vi "GeoData.vi"() -> ()   [LabVIEW 2017] (continued)
County\tH1\n52577\t19123\tOskaloosa\tIA\tMahaska County\tH1\n50256\t19123\tTracy\tIA\tMahaska County\tH1\n52595\t19123\tUniversity park\tIA\tMahaska County\tH1\n50207\t19123\tNew sharon\tIA\tMahaska County\tH1\n50027\t19123\tBarnes city\tIA\tMahaska County\tH1\n50170\t19125\tMonroe\tIA\tMarion County\tH1\n50163\t19125\tMelcher dallas\tIA\tMarion County\tH1\n50049\t19125\tChariton\tIA\tMarion County\tH1\n50138\t19125\tKnoxville\tIA\tMarion County\tH1\n50219\t19125\tPella\tIA\tMarion County\tH1\n50214\t19125\tOtley\tIA\tMarion County\tH1\n50143\t19125\tLeighton\tIA\tMarion County\tH1\n50237\t19125\tRunnells\tIA\tMarion County\tH1\n50252\t19125\tSwan\tIA\tMarion County\tH1\n50228\t19125\tPrairie city\tIA\tMarion County\tH1\n50139\t19125\tLacona\tIA\tMarion County\tH1\n50044\t19125\tBussey\tIA\tMarion County\tH1\n50150\t19125\tLovilia\tIA\tMarion County\tH1\n50062\t19125\tMelcher dallas\tIA\tMarion County\tH1\n50256\t19125\tTracy\tIA\tMarion County\tH1\n50057\t19125\tColumbia\tIA\tMarion County\tH1\n50119\t19125\tHarvey\tIA\tMarion County\tH1\n50225\t19125\tPleasantville\tIA\tMarion County\tH1\n50116\t19125\tHamilton\tIA\tMarion County\tH1\n50206\t19127\tNew providence\tIA\tMarshall County\tH1\n50632\t19127\tGarwin\tIA\tMarshall County\tH1\n50078\t19127\tFerguson\tIA\tMarshall County\tH1\n50239\t19127\tSaint anthony\tIA\tMarshall County\tH1\n50120\t19127\tHaverhill\tIA\tMarshall County\tH1\n50148\t19127\tLiscomb\tIA\tMarshall County\tH1\n50621\t19127\tConrad\tIA\tMarshall County\tH1\n50173\t19127\tMontour\tIA\tMarshall County\tH1\n50051\t19127\tClemons\tIA\tMarshall County\tH1\n50158\t19127\tMarshalltown\tIA\tMarshall County\tH1\n50141\t19127\tLaurel\tIA\tMarshall County\tH1\n50609\t19127\tBeaman\tIA\tMarshall County\tH1\n50234\t19127\tRhodes\tIA\tMarshall County\tH1\n50247\t19127\tState center\tIA\tMarshall County\tH1\n50162\t19127\tMelbourne\tIA\tMarshall County\tH1\n50635\t19127\tGladbrook\tIA\tMarshall County\tH1\n50005\t19127\tAlbion\tIA\tMarshall County\tH1\n50142\t19127\tLe grand\tIA\tMarshall County\tH1\n50055\t19127\tCollins\tIA\tMarshall County\tH1\n50258\t19127\tUnion\tIA\tMarshall County\tH1\n50028\t19127\tBaxter\tIA\tMarshall County\tH1\n50106\t19127\tGilman\tIA\tMarshall County\tH1\n51551\t19129\tMalvern\tIA\tMills County\tH1\n51541\t19129\tHenderson\tIA\tMills County\tH1\n51571\t19129\tSilver city\tIA\tMills County\tH1\n51540\t19129\tHastings\tIA\tMills County\tH1\n51533\t19129\tEmerson\tIA\tMills County\tH1\n51534\t19129\tGlenwood\tIA\tMills County\tH1\n51653\t19129\tTabor\tIA\tMills County\tH1\n51503\t19129\tCouncil bluffs\tIA\tMills County\tH1\n51554\t19129\tMineola\tIA\tMills County\tH1\n51549\t19129\tMacedonia\tIA\tMills County\tH1\n51561\t19129\tPacific junction\tIA\tMills County\tH1\n51645\t19129\tImogene\tIA\tMills County\tH1\n50458\t19131\tNora springs\tIA\tMitchell County\tH1\n50464\t19131\tPlymouth\tIA\tMitchell County\tH1\n50426\t19131\tCarpenter\tIA\tMitchell County\tH1\n50461\t19131\tOsage\tIA\tMitchell County\tH1\n50628\t19131\tElma\tIA\tMitchell County\tH1\n50481\t19131\tToeterville\tIA\tMitchell County\tH1\n50472\t19131\tSaint ansgar\tIA\tMitchell County\tH1\n50471\t19131\tRudd\tIA\tMitchell County\tH1\n50603\t19131\tAlta vista\tIA\tMitchell County\tH1\n50466\t19131\tRiceville\tIA\tMitchell County\tH1\n50455\t19131\tMc intire\tIA\tMitchell County\tH1\n50476\t19131\tStacyville\tIA\tMitchell County\tH1\n50435\t19131\tFloyd\tIA\tMitchell County\tH1\n50460\t19131\tOrchard\tIA\tMitchell County\tH1\n50454\t19131\tLittle cedar\tIA\tMitchell County\tH1\n51572\t19133\tSoldier\tIA\tMonona County\tH1\n51056\t19133\tSmithland\tIA\tMonona County\tH1\n51545\t19133\tLittle sioux\tIA\tMonona County\tH1\n51026\t19133\tHornick\tIA\tMonona County\tH1\n51063\t19133\tWhiting\tIA\tMonona County\tH1\n51040\t19133\tOnawa\tIA\tMonona County\tH1\n51055\t19133\tSloan\tIA\tMonona County\tH1\n51034\t19133\tMapleton\tIA\tMonona County\tH1\n51523\t19133\tBlencoe\tIA\tMonona County\tH1\n51529\t19133\tDunlap\tIA\tMonona County\tH1\n51010\t19133\tCastana\tIA\tMonona County\tH1\n51019\t19133\tDanbury\tIA\tMonona County\tH1\n51060\t19133\tUte\tIA\tMonona County\tH1\n51051\t19133\tRodney\tIA\tMonona County\tH1\n51558\t19133\tMoorhead\tIA\tMonona County\tH1\n52553\t19135\tEddyville\tIA\tMonroe County\tH1\n50044\t19135\tBussey\tIA\tMonroe County\tH1\n50150\t19135\tLovilia\tIA\tMonroe County\tH1\n52536\t19135\tBlakesburg\tIA\tMonroe County\tH1\n52571\t19135\tMoravia\tIA\tMonroe County\tH1\n52531\t19135\tAlbia\tIA\tMonroe County\tH1\n52569\t19135\tMelrose\tIA\tMonroe County\tH1\n52594\t19135\tUnionville\tIA\tMonroe County\tH1\n50857\t19137\tNodaway\tIA\tMontgomery County\tH1\n51532\t19137\tElliott\tIA\tMontgomery County\tH1\n50847\t19137\tGrant\tIA\tMontgomery County\tH1\n51541\t19137\tHenderson\tIA\tMontgomery County\tH1\n51638\t19137\tEssex\tIA\tMontgomery County\tH1\n51573\t19137\tStanton\tIA\tMontgomery County\tH1\n50843\t19137\tCumberland\tIA\tMontgomery County\tH1\n51533\t19137\tEmerson\tIA\tMontgomery County\tH1\n50841\t19137\tCorning\tIA\tMontgomery County\tH1\n50864\t19137\tVillisca\tIA\tMontgomery County\tH1\n51549\t19137\tMacedonia\tIA\tMontgomery County\tH1\n51566\t19137\tRed oak\tIA\tMontgomery County\tH1\n51645\t19137\tImogene\tIA\tMontgomery County\tH1\n52720\t19139\tAtalissa\tIA\tMuscatine County\tH1\n52726\t19139\tBlue grass\tIA\tMuscatine County\tH1\n52776\t19139\tWest liberty\tIA\tMuscatine County\tH1\n52759\t19139\tMontpelier\tIA\tMuscatine County\tH1\n52761\t19139\tMuscatine\tIA\tMuscatine County\tH1\n52739\t19139\tConesville\tIA\tMuscatine County\tH1\n52747\t19139\tDurant\tIA\tMuscatine County\tH1\n52766\t19139\tNichols\tIA\tMuscatine County\tH1\n52754\t19139\tLetts\tIA\tMuscatine County\tH1\n52755\t19139\tLone tree\tIA\tMuscatine County\tH1\n52749\t19139\tFruitland\tIA\tMuscatine County\tH1\n52778\t19139\tWilton\tIA\tMuscatine County\tH1\n52760\t19139\tMoscow\tIA\tMuscatine County\tH1\n52773\t19139\tWalcott\tIA\tMuscatine County\tH1\n52769\t19139\tStockton\tIA\tMuscatine County\tH1\n51201\t19141\tSheldon\tIA\tO'Brien County\tH1\n51047\t19141\tPeterson\tIA\tO'Brien County\tH1\n51046\t19141\tPaullina\tIA\tO'Brien County\tH1\n51248\t19141\tSanborn\tIA\tO'Brien County\tH1\n51350\t19141\tMelvin\tIA\tO'Brien County\tH1\n51346\t19141\tHartley\tIA\tO'Brien County\tH1\n51231\t19141\tArcher\tIA\tO'Brien County\tH1\n51035\t19141\tMarcus\tIA\tO'Brien County\tH1\n51238\t19141\tHospers\tIA\tO'Brien County\tH1\n51014\t19141\tCleghorn\tIA\tO'Brien County\tH1\n51029\t19141\tLarrabee\tIA\tO'Brien County\tH1\n51009\t19141\tCalumet\tIA\tO'Brien County\tH1\n51022\t19141\tGranville\tIA\tO'Brien County\tH1\n51245\t19141\tPrimghar\tIA\tO'Brien County\tH1\n51232\t19141\tAshton\tIA\tO'Brien County\tH1\n51058\t19141\tSutherland\tIA\tO'Brien County\tH1\n51201\t19143\tSheldon\tIA\tOsceola County\tH1\n51347\t19143\tLake park\tIA\tOsceola County\tH1\n51248\t19143\tSanborn\tIA\tOsceola County\tH1\n51243\t19143\tLittle rock\tIA\tOsceola County\tH1\n51350\t19143\tMelvin\tIA\tOsceola County\tH1\n51346\t19143\tHartley\tIA\tOsceola County\tH1\n51354\t19143\tOcheyedan\tIA\tOsceola County\tH1\n51345\t19143\tHarris\tIA\tOsceola County\tH1\n51249\t19143\tSibley\tIA\tOsceola County\tH1\n51232\t19143\tAshton\tIA\tOsceola County\tH1\n51647\t19145\tNorthboro\tIA\tPage County\tH1\n51656\t19145\tYorktown\tIA\tPage County\tH1\n51638\t19145\tEssex\tIA\tPage County\tH1\n51651\t19145\tShambaugh\tIA\tPage County\tH1\n51603\t19145\tShenandoah\tIA\tPage County\tH1\n51601\t19145\tShenandoah\tIA\tPage County\tH1\n50864\t19145\tVillisca\tIA\tPage County\tH1\n51630\t19145\tBlanchard\tIA\tPage County\tH1\n51632\t19145\tClarinda\tIA\tPage County\tH1\n51636\t19145\tCoin\tIA\tPage County\tH1\n51646\t19145\tNew market\tIA\tPage County\tH1\n51631\t19145\tBraddyville\tIA\tPage County\tH1\n50833\t19145\tBedford\tIA\tPage County\tH1\n51566\t19145\tRed oak\tIA\tPage County\tH1\n51637\t19145\tCollege springs\tIA\tPage County\tH1\n51645\t19145\tImogene\tIA\tPage County\tH1\n50546\t19147\tHavelock\tIA\tPalo Alto County\tH1\n50581\t19147\tRolfe\tIA\tPalo Alto County\tH1\n50554\t19147\tLaurens\tIA\tPalo Alto County\tH1\n50562\t19147\tMallard\tIA\tPalo Alto County\tH1\n50578\t19147\tRingsted\tIA\tPalo Alto County\tH1\n51342\t19147\tGraettinger\tIA\tPalo Alto County\tH1\n51358\t19147\tRuthven\tIA\tPalo Alto County\tH1\n50539\t19147\tFenton\tIA\tPalo Alto County\tH1\n51366\t19147\tWebb\tIA\tPalo Alto County\tH1\n50515\t19147\tAyrshire\tIA\tPalo Alto County\tH1\n50528\t19147\tCylinder\tIA\tPalo Alto County\tH1\n50536\t19147\tEmmetsburg\tIA\tPalo Alto County\tH1\n51364\t19147\tTerril\tIA\tPalo Alto County\tH1\n50527\t19147\tCurlew\tIA\tPalo Alto County\tH1\n50598\t19147\tWhittemore\tIA\tPalo Alto County\tH1\n50597\t19147\tWest bend\tIA\tPalo Alto County\tH1\n51109\t19149\tSioux city\tIA\tPlymouth County\tH1\n51108\t19149\tSioux city\tIA\tPlymouth County\tH1\n51048\t19149\tPierson\tIA\tPlymouth County\tH1\n51027\t19149\tIreton\tIA\tPlymouth County\tH1\n51001\t19149\tAkron\tIA\tPlymouth County\tH1\n51024\t19149\tHinton\tIA\tPlymouth County\tH1\n51028\t19149\tKingsley\tIA\tPlymouth County\tH1\n51035\t19149\tMarcus\tIA\tPlymouth County\tH1\n51062\t19149\tWestfield\tIA\tPlymouth County\tH1\n51036\t19149\tMaurice\tIA\tPlymouth County\tH1\n51008\t19149\tBrunsville\tIA\tPlymouth County\tH1\n51050\t19149\tRemsen\tIA\tPlymouth County\tH1\n51041\t19149\tOrange city\tIA\tPlymouth County\tH1\n51031\t19149\tLe mars\tIA\tPlymouth County\tH1\n51003\t19149\tAlton\tIA\tPlymouth County\tH1\n51038\t19149\tMerrill\tIA\tPlymouth County\tH1\n51023\t19149\tHawarden\tIA\tPlymouth County\tH1\n51022\t19149\tGranville\tIA\tPlymouth County\tH1\n51045\t19149\tOyens\tIA\tPlymouth County\tH1\n50568\t19151\tNewell\tIA\tPocahontas County\tH1\n50546\t19151\tHavelock\tIA\tPocahontas County\tH1\n50593\t19151\tVarina\tIA\tPocahontas County\tH1\n50581\t19151\tRolfe\tIA\tPocahontas County\tH1\n50554\t19151\tLaurens\tIA\tPocahontas County\tH1\n50562\t19151\tMallard\tIA\tPocahontas County\tH1\n50571\t19151\tPalmer\tIA\tPocahontas County\tH1\n50540\t19151\tFonda\tIA\tPocahontas County\tH1\n50573\t19151\tPlover\tIA\tPocahontas County\tH1\n50510\t19151\tAlbert city\tIA\tPocahontas County\tH1\n50574\t19151\tPocahontas\tIA\tPocahontas County\tH1\n50520\t19151\tBradgate\tIA\tPocahontas County\tH1\n50541\t19151\tGilmore city\tIA\tPocahontas County\tH1\n50524\t19151\tClare\tIA\tPocahontas County\tH1\n50563\t19151\tManson\tIA\tPocahontas County\tH1\n50575\t19151\tPomeroy\tIA\tPocahontas County\tH1\n50597\t19151\tWest bend\tIA\tPocahontas County\tH1\n50109\t19153\tGranger\tIA\tPolk County\tH1\n50318\t19153\tDes moines\tIA\tPolk County\tH1\n50009\t19153\tAltoona\tIA\tPolk County\tH1\n50319\t19153\tDes moines\tIA\tPolk County\tH1\n50032\t19153\tBerwick\tIA\tPolk County\tH1\n50364\t19153\tDes moines\tIA\tPolk County\tH1\n50169\t19153\tMitchellville\tIA\tPolk County\tH1\n50244\t19153\tSlater\tIA\tPolk County\tH1\n50313\t19153\tDes moines\tIA\tPolk County\tH1\n50314\t19153\tDes moines\tIA\tPolk County\tH1\n50317\t19153\tDes moines\tIA\tPolk County\tH1\n50391\t19153\tDes moines\tIA\tPolk County\tH1\n50324\t19153\tWindsor heights\tIA\tPolk County\tH1\n50302\t19153\tDes moines\tIA\tPolk County\tH1\n50304\t19153\tDes moines\tIA\tPolk County\tH1\n50362\t19153\tDes moines\tIA\tPolk County\tH1\n50380\t19153\tDes moines\tIA\tPolk County\tH1\n50161\t19153\tMaxwell\tIA\tPolk County\tH1\n50046\t19153\tCambridge\tIA\tPolk County\tH1\n50035\t19153\tBondurant\tIA\tPolk County\tH1\n50054\t19153\tColfax\tIA\tPolk County\tH1\n50237\t19153\tRunnells\tIA\tPolk County\tH1\n50316\t19153\tDes moines\tIA\tPolk County\tH1\n50320\t19153\tDes moines\tIA\tPolk County\tH1\n50395\t19153\tDes moines\tIA\tPolk County\tH1\n50363\t19153\tDes moines\tIA\tPolk County\tH1\n50368\t19153\tDes moines\tIA\tPolk County\tH1\n50359\t19153\tDes moines\tIA\tPolk County\tH1\n50361\t19153\tDes moines\tIA\tPolk County\tH1\n50328\t19153\tDes moines\tIA\tPolk County\tH1\n50061\t19153\tCumming\tIA\tPolk County\tH1\n50325\t19153\tClive\tIA\tPolk County\tH1\n50265\t19153\tWest des moines\tIA\tPolk County\tH1\n50327\t19153\tPleasant hill\tIA\tPolk County\tH1\n50007\t19153\tAlleman\tIA\tPolk County\tH1\n50168\t19153\tMingo\tIA\tPolk County\tH1\n50301\t19153\tDes moines\tIA\tPolk County\tH1\n50360\t19153\tDes moines\tIA\tPolk County\tH1\n50023\t19153\tAnkeny\tIA\tPolk County\tH1\n50228\t19153\tPrairie city\tIA\tPolk County\tH1\n50226\t19153\tPolk city\tIA\tPolk County\tH1\n50311\t19153\tDes moines\tIA\tPolk County\tH1\n50312\t19153\tDes moines\tIA\tPolk County\tH1\n50156\t19153\tMadrid\tIA\tPolk County\tH1\n50131\t19153\tJohnston\tIA\tPolk County\tH1\n50315\t19153\tDes moines\tIA\tPolk County\tH1\n50310\t19153\tDes moines\tIA\tPolk County\tH1\n50305\t19153\tDes moines\tIA\tPolk County\tH1\n50303\t19153\tDes moines\tIA\tPolk County\tH1\n50111\t19153\tGrimes\tIA\tPolk County\tH1\n50047\t19153\tCarlisle\tIA\tPolk County\tH1\n50323\t19153\tUrbandale\tIA\tPolk County\tH1\n50243\t19153\tSheldahl\tIA\tPolk County\tH1\n50392\t19153\tDes moines\tIA\tPolk County\tH1\n50398\t19153\tUrbandale\tIA\tPolk County\tH1\n50021\t19153\tAnkeny\tIA\tPolk County\tH1\n50073\t19153\tElkhart\tIA\tPolk County\tH1\n50322\t19153\tUrbandale\tIA\tPolk County\tH1\n50266\t19153\tWest des moines\tIA\tPolk County\tH1\n50321\t19153\tDes moines\tIA\tPolk County\tH1\n50309\t19153\tDes moines\tIA\tPolk County\tH1\n50124\t19153\tHuxley\tIA\tPolk County\tH1\n50947\t19153\tDes moines\tIA\tPolk County\tH1\n51525\t19155\tCarson\tIA\tPottawattamie County\tH1\n51576\t19155\tUnderwood\tIA\tPottawattamie County\tH1\n51532\t19155\tElliott\tIA\tPottawattamie County\tH1\n51560\t19155\tOakland\tIA\tPottawattamie County\tH1\n51541\t19155\tHenderson\tIA\tPottawattamie County\tH1\n51571\t19155\tSilver city\tIA\tPottawattamie County\tH1\n51548\t19155\tMc clelland\tIA\tPottawattamie County\tH1\n51553\t19155\tMinden\tIA\tPottawattamie County\tH1\n51501\t19155\tCouncil bluffs\tIA\tPottawattamie County\tH1\n51521\t19155\tAvoca\tIA\tPottawattamie County\tH1\n51536\t19155\tHancock\tIA\tPottawattamie County\tH1\n51552\t19155\tMarne\tIA\tPottawattamie County\tH1\n51555\t19155\tMissouri valley\tIA\tPottawattamie County\tH1\n51542\t19155\tHoney creek\tIA\tPottawattamie County\tH1\n51544\t19155\tLewis\tIA\tPottawattamie County\tH1\n51577\t19155\tWalnut\tIA\tPottawattamie County\tH1\n51503\t19155\tCouncil bluffs\tIA\tPottawattamie County\tH1\n51575\t19155\tTreynor\tIA\tPottawattamie County\tH1\n51502\t19155\tCouncil bluffs\tIA\tPottawattamie County\tH1\n51526\t19155\tCrescent\tIA\tPottawattamie County\tH1\n51510\t19155\tCarter lake\tIA\tPottawattamie County\tH1\n51559\t19155\tNeola\tIA\tPottawattamie County\tH1\n51549\t19155\tMacedonia\tIA\tPottawattamie County\tH1\n51566\t19155\tRed oak\tIA\tPottawattamie County\tH1\n51535\t19155\tGriswold\tIA\tPottawattamie County\tH1\n51570\t19155\tShelby\tIA\tPottawattamie County\tH1\n52339\t19157\tTama\tIA\tPoweshiek County\tH1\n50153\t19157\tLynnville\tIA\tPoweshiek County\tH1\n50104\t19157\tGibson\tIA\tPoweshiek County\tH1\n50157\t19157\tMalcom\tIA\tPoweshiek County\tH1\n52232\t19157\tHartwick\tIA\tPoweshiek County\tH1\n52215\t19157\tChelsea\tIA\tPoweshiek County\tH1\n50171\t19157\tMontezuma\tIA\tPoweshiek County\tH1\n52222\t19157\tDeep river\tIA\tPoweshiek County\tH1\n52347\t19157\tVictor\tIA\tPoweshiek County\tH1\n50112\t19157\tGrinnell\tIA\tPoweshiek County\tH1\n52221\t19157\tGuernsey\tIA\tPoweshiek County\tH1\n52211\t19157\tBrooklyn\tIA\tPoweshiek County\tH1\n52208\t19157\tBelle plaine\tIA\tPoweshiek County\tH1\n50207\t19157\tNew sharon\tIA\tPoweshiek County\tH1\n50106\t19157\tGilman\tIA\tPoweshiek County\tH1\n50242\t19157\tSearsboro\tIA\tPoweshiek County\tH1\n50027\t19157\tBarnes city\tIA\tPoweshiek County\tH1\n50861\t19159\tShannon city\tIA\tRinggold County\tH1\n50860\t19159\tRedding\tIA\tRinggold County\tH1\n50074\t19159\tEllston\tIA\tRinggold County\tH1\n50140\t19159\tLamoni\tIA\tRinggold County\tH1\n50863\t19159\tTingley\tIA\tRinggold County\tH1\n50840\t19159\tClearfield\tIA\tRinggold County\tH1\n50845\t19159\tDiagonal\tIA\tRinggold County\tH1\n50133\t19159\tKellerton\tIA\tRinggold County\tH1\n50854\t19159\tMount ayr\tIA\tRinggold County\tH1\n50851\t19159\tLenox\tIA\tRinggold County\tH1\n50836\t19159\tBlockton\tIA\tRinggold County\tH1\n50835\t19159\tBenton\tIA\tRinggold County\tH1\n50568\t19161\tNewell\tIA\tSac County\tH1\n51458\t19161\tOdebolt\tIA\tSac County\tH1\n51450\t19161\tLake view\tIA\tSac County\tH1\n51466\t19161\tWall lake\tIA\tSac County\tH1\n50567\t19161\tNemaha\tIA\tSac County\tH1\n51020\t19161\tGalva\tIA\tSac County\tH1\n51433\t19161\tAuburn\tIA\tSac County\tH1\n50561\t19161\tLytton\tIA\tSac County\tH1\n50540\t19161\tFonda\tIA\tSac County\tH1\n51431\t19161\tArthur\tIA\tSac County\tH1\n51002\t19161\tAlta\tIA\tSac County\tH1\n51053\t19161\tSchaller\tIA\tSac County\tH1\n50583\t19161\tSac city\tIA\tSac County\tH1\n50588\t19161\tStorm lake\tIA\tSac County\tH1\n51448\t19161\tKiron\tIA\tSac County\tH1\n50535\t19161\tEarly\tIA\tSac County\tH1\n51436\t19161\tBreda\tIA\tSac County\tH1\n52748\t19163\tEldridge\tIA\tScott County\tH1\n52809\t19163\tDavenport\tIA\tScott County\tH1\n52804\t19163\tDavenport\tIA\tScott County\tH1\n52726\t19163\tBlue grass\tIA\tScott County\tH1\n52808\t19163\tDavenport\tIA\tScott County\tH1\n52767\t19163\tPleasant valley\tIA\tScott County\tH1\n52806\t19163\tDavenport\tIA\tScott County\tH1\n52801\t19163\tDavenport\tIA\tScott County\tH1\n52768\t19163\tPrinceton\tIA\tScott County\tH1\n52759\t19163\tMontpelier\tIA\tScott County\tH1\n52803\t19163\tDavenport\tIA\tScott County\tH1\n52807\t19163\tDavenport\tIA\tScott County\tH1\n52745\t19163\tDixon\tIA\tScott County\tH1\n52747\t19163\tDurant\tIA\tScott County\tH1\n52765\t19163\tNew liberty\tIA\tScott County\tH1\n52722\t19163\tBettendorf\tIA\tScott County\tH1\n52802\t19163\tDavenport\tIA\tScott County\tH1\n52756\t19163\tLong grove\tIA\tScott County\tH1\n52758\t19163\tMc causland\tIA\tScott County\tH1\n52753\t19163\tLe claire\tIA\tScott County\tH1\n52773\t19163\tWalcott\tIA\tScott County\tH1\n52746\t19163\tDonahue\tIA\tScott County\tH1\n52769\t19163\tStockton\tIA\tScott County\tH1\n52728\t19163\tBuffalo\tIA\tScott County\tH1\n52805\t19163\tDavenport\tIA\tScott County\tH1\n51578\t19165\tWestphalia\tIA\tShelby County\tH1\n50076\t19165\tExira\tIA\tShelby County\tH1\n51447\t19165\tKirkman\tIA\tShelby County\tH1\n51527\t19165\tDefiance\tIA\tShelby County\tH1\n51563\t19165\tPersia\tIA\tShelby County\tH1\n51531\t19165\tElk horn\tIA\tShelby County\tH1\n51455\t19165\tManning\tIA\tShelby County\tH1\n51521\t19165\tAvoca\tIA\tShelby County\tH1\n51552\t19165\tMarne\tIA\tShelby County\tH1\n51446\t19165\tIrwin\tIA\tShelby County\tH1\n51562\t19165\tPanama\tIA\tShelby County\tH1\n51529\t19165\tDunlap\tIA\tShelby County\tH1\n51565\t19165\tPortsmouth\tIA\tShelby County\tH1\n50022\t19165\tAtlantic\tIA\tShelby County\tH1\n51454\t19165\tManilla\tIA\tShelby County\tH1\n51577\t19165\tWalnut\tIA\tShelby County\tH1\n51528\t19165\tDow city\tIA\tShelby County\tH1\n50025\t19165\tAudubon\tIA\tShelby County\tH1\n51543\t19165\tKimballton\tIA\tShelby County\tH1\n51537\t19165\tHarlan\tIA\tShelby County\tH1\n51530\t19165\tEarling\tIA\tShelby County\tH1\n51570\t19165\tShelby\tIA\tShelby County\tH1\n51201\t19167\tSheldon\tIA\tSioux County\tH1\n51011\t19167\tChatsworth\tIA\tSioux County\tH1\n51027\t19167\tIreton\tIA\tSioux County\tH1\n51234\t19167\tBoyden\tIA\tSioux County\tH1\n51235\t19167\tDoon\tIA\tSioux County\tH1\n51238\t19167\tHospers\tIA\tSioux County\tH1\n51036\t19167\tMaurice\tIA\tSioux County\tH1\n51050\t19167\tRemsen\tIA\tSioux County\tH1\n51041\t19167\tOrange city\tIA\tSioux County\tH1\n51031\t19167\tLe mars\tIA\tSioux County\tH1\n51003\t19167\tAlton\tIA\tSioux County\tH1\n51239\t19167\tHull\tIA\tSioux County\tH1\n51247\t19167\tRock valley\tIA\tSioux County\tH1\n51240\t19167\tInwood\tIA\tSioux County\tH1\n51023\t19167\tHawarden\tIA\tSioux County\tH1\n51244\t19167\tMatlock\tIA\tSioux County\tH1\n51022\t19167\tGranville\tIA\tSioux County\tH1\n51250\t19167\tSioux center\tIA\tSioux County\tH1\n51232\t19167\tAshton\tIA\tSioux County\tH1\n50201\t19169\tNevada\tIA\tStory County\tH1\n50206\t19169\tNew providence\tIA\tStory County\tH1\n50236\t19169\tRoland\tIA\tStory County\tH1\n50105\t19169\tGilbert\tIA\tStory County\tH1\n50239\t19169\tSaint anthony\tIA\tStory County\tH1\n50014\t19169\tAmes\tIA\tStory County\tH1\n50056\t19169\tColo\tIA\tStory County\tH1\n50230\t19169\tRadcliffe\tIA\tStory County\tH1\n50244\t19169\tSlater\tIA\tStory County\tH1\n50278\t19169\tZearing\tIA\tStory County\tH1\n50134\t19169\tKelley\tIA\tStory County\tH1\n50011\t19169\tAmes\tIA\tStory County\tH1\n50013\t19169\tAmes\tIA\tStory County\tH1\n50161\t19169\tMaxwell\tIA\tStory County\tH1\n50010\t19169\tAmes\tIA\tStory County\tH1\n50046\t19169\tCambridge\tIA\tStory County\tH1\n50122\t19169\tHubbard\tIA\tStory County\tH1\n50226\t19169\tPolk city\tIA\tStory County\tH1\n50012\t19169\tAmes\tIA\tStory County\tH1\n50247\t19169\tState center\tIA\tStory County\tH1\n50248\t19169\tStory city\tIA\tStory County\tH1\n50243\t19169\tSheldahl\tIA\tStory County\tH1\n50055\t19169\tCollins\tIA\tStory County\tH1\n50154\t19169\tMc callsburg\tIA\tStory County\tH1\n50124\t19169\tHuxley\tIA\tStory County\tH1\n50638\t19171\tGrundy center\tIA\tTama County\tH1\n50651\t19171\tLa porte city\tIA\tTama County\tH1\n50632\t19171\tGarwin\tIA\tTama County\tH1\n52339\t19171\tTama\tIA\tTama County\tH1\n50652\t19171\tLincoln\tIA\tTama County\tH1\n52342\t19171\tToledo\tIA\tTama County\tH1\n52225\t19171\tElberon\tIA\tTama County\tH1\n50173\t19171\tMontour\tIA\tTama County\tH1\n52215\t19171\tChelsea\tIA\tTama County\tH1\n52348\t19171\tVining\tIA\tTama County\tH1\n50669\t19171\tReinbeck\tIA\tTama County\tH1\n52217\t19171\tClutier\tIA\tTama County\tH1\n50158\t19171\tMarshalltown\tIA\tTama County\tH1\n50609\t19171\tBeaman\tIA\tTama County\tH1\n52224\t19171\tDysart\tIA\tTama County\tH1\n50635\t19171\tGladbrook\tIA\tTama County\tH1\n52208\t19171\tBelle plaine\tIA\tTama County\tH1\n50675\t19171\tTraer\tIA\tTama County\tH1\n50106\t19171\tGilman\tIA\tTama County\tH1\n50612\t19171\tBuckingham\tIA\tTama County\tH1\n50857\t19173\tNodaway\tIA\tTaylor County\tH1\n50862\t19173\tSharpsburg\tIA\tTaylor County\tH1\n50841\t19173\tCorning\tIA\tTaylor County\tH1\n50864\t19173\tVillisca\tIA\tTaylor County\tH1\n50840\t19173\tClearfield\tIA\tTaylor County\tH1\n51632\t19173\tClarinda\tIA\tTaylor County\tH1\n50848\t19173\tGravity\tIA\tTaylor County\tH1\n51646\t19173\tNew market\tIA\tTaylor County\tH1\n50833\t19173\tBedford\tIA\tTaylor County\tH1\n50851\t19173\tLenox\tIA\tTaylor County\tH1\n50836\t19173\tBlockton\tIA\tTaylor County\tH1\n50861\t19175\tShannon city\tIA\tUnion County\tH1\n50830\t19175\tAfton\tIA\tUnion County\tH1\n50074\t19175\tEllston\tIA\tUnion County\tH1\n50254\t19175\tThayer\tIA\tUnion County\tH1\n50801\t19175\tCreston\tIA\tUnion County\tH1\n50842\t19175\tCromwell\tIA\tUnion County\tH1\n50149\t19175\tLorimor\tIA\tUnion County\tH1\n50845\t19175\tDiagonal\tIA\tUnion County\tH1\n50831\t19175\tArispe\tIA\tUnion County\tH1\n50851\t19175\tLenox\tIA\tUnion County\tH1\n50174\t19175\tMurray\tIA\tUnion County\tH1\n52570\t19177\tMilton\tIA\tVan Buren County\tH1\n52620\t19177\tBonaparte\tIA\tVan Buren County\tH1\n52630\t19177\tHillsboro\tIA\tVan Buren County\tH1\n52573\t19177\tMount sterling\tIA\tVan Buren County\tH1\n52584\t19177\tPulaski\tIA\tVan Buren County\tH1\n52551\t19177\tDouds\tIA\tVan Buren County\tH1\n52626\t19177\tFarmington\tIA\tVan Buren County\tH1\n52567\t19177\tLibertyville\tIA\tVan Buren County\tH1\n52588\t19177\tSelma\tIA\tVan Buren County\tH1\n52565\t19177\tKeosauqua\tIA\tVan Buren County\tH1\n52542\t19177\tCantril\tIA\tVan Buren County\tH1\n52554\t19177\tEldon\tIA\tVan Buren County\tH1\n52535\t19177\tBirmingham\tIA\tVan Buren County\tH1\n52651\t19177\tStockport\tIA\tVan Buren County\tH1\n52553\t19179\tEddyville\tIA\tWapello County\tH1\n52566\t19179\tKirkville\tIA\tWapello County\tH1\n52533\t19179\tBatavia\tIA\tWapello County\tH1\n52563\t19179\tHedrick\tIA\tWapello County\tH1\n52561\t19179\tFremont\tIA\tWapello County\tH1\n52501\t19179\tOttumwa\tIA\tWapello County\tH1\n52530\t19179\tAgency\tIA\tWapello County\tH1\n52548\t19179\tChillicothe\tIA\tWapello County\tH1\n52552\t19179\tDrakesville\tIA\tWapello County\tH1\n52536\t19179\tBlakesburg\tIA\tWapello County\tH1\n52554\t19179\tEldon\tIA\tWapello County\tH1\n52531\t19179\tAlbia\tIA\tWapello County\tH1\n52537\t19179\tBloomfield\tIA\tWapello County\tH1\n50125\t19181\tIndianola\tIA\tWarren County\tH1\n50001\t19181\tAckworth\tIA\tWarren County\tH1\n50257\t19181\tTruro\tIA\tWarren County\tH1\n50118\t19181\tHartford\tIA\tWarren County\tH1\n50229\t19181\tProle\tIA\tWarren County\tH1\n50240\t19181\tSaint charles\tIA\tWarren County\tH1\n50320\t19181\tDes moines\tIA\tWarren County\tH1\n50145\t19181\tLiberty center\tIA\tWarren County\tH1\n50061\t19181\tCumming\tIA\tWarren County\tH1\n50265\t19181\tWest des moines\tIA\tWarren County\tH1\n50252\t19181\tSwan\tIA\tWarren County\tH1\n50213\t19181\tOsceola\tIA\tWarren County\tH1\n50139\t19181\tLacona\tIA\tWarren County\tH1\n50160\t19181\tMartensdale\tIA\tWarren County\tH1\n50211\t19181\tNorwalk\tIA\tWarren County\tH1\n50151\t19181\tLucas\tIA\tWarren County\tH1\n50241\t19181\tSaint marys\tIA\tWarren County\tH1\n50047\t19181\tCarlisle\tIA\tWarren County\tH1\n50225\t19181\tPleasantville\tIA\tWarren County\tH1\n50033\t19181\tBevington\tIA\tWarren County\tH1\n50166\t19181\tMilo\tIA\tWarren County\tH1\n50210\t19181\tNew virginia\tIA\tWarren County\tH1\n50321\t19181\tDes moines\tIA\tWarren County\tH1\n52247\t19183\tKalona\tIA\tWashington County\tH1\n52641\t19183\tMount pleasant\tIA\tWashington County\tH1\n52585\t19183\tRichland\tIA\tWashington County\tH1\n52621\t19183\tCrawfordsville\tIA\tWashington County\tH1\n52353\t19183\tWashington\tIA\tWashington County\tH1\n52540\t19183\tBrighton\tIA\tWashington County\tH1\n52738\t19183\tColumbus junction\tIA\tWashington County\tH1\n52359\t19183\tWest chester\tIA\tWashington County\tH1\n52201\t19183\tAinsworth\tIA\tWashington County\tH1\n52356\t19183\tWellman\tIA\tWashington County\tH1\n52248\t19183\tKeota\tIA\tWashington County\tH1\n52327\t19183\tRiverside\tIA\tWashington County\tH1\n52654\t19183\tWayland\tIA\tWashington County\tH1\n50060\t19185\tCorydon\tIA\tWayne County\tH1\n50049\t19185\tChariton\tIA\tWayne County\tH1\n50147\t19185\tLineville\tIA\tWayne County\tH1\n50238\t19185\tRussell\tIA\tWayne County\tH1\n52581\t19185\tPlano\tIA\tWayne County\tH1\n50123\t19185\tHumeston\tIA\tWayne County\tH1\n50052\t19185\tClio\tIA\tWayne County\tH1\n50068\t19185\tDerby\tIA\tWayne County\tH1\n50103\t19185\tGarden grove\tIA\tWayne County\tH1\n50008\t19185\tAllerton\tIA\tWayne County\tH1\n52583\t19185\tPromise city\tIA\tWayne County\tH1\n52590\t19185\tSeymour\tIA\tWayne County\tH1\n52569\t19185\tMelrose\tIA\tWayne County\tH1\n50165\t19185\tMillerton\tIA\tWayne County\tH1\n50530\t19187\tDayton\tIA\tWebster County\tH1\n50543\t19187\tGowrie\tIA\tWebster County\tH1\n50594\t19187\tVincent\tIA\tWebster County\tH1\n50586\t19187\tSomers\tIA\tWebster County\tH1\n50518\t19187\tBarnum\tIA\tWebster County\tH1\n50548\t19187\tHumboldt\tIA\tWebster County\tH1\n50595\t19187\tWebster city\tIA\tWebster County\tH1\n50516\t19187\tBadger\tIA\tWebster County\tH1\n50501\t19187\tFort dodge\tIA\tWebster County\tH1\n50521\t19187\tBurnside\tIA\tWebster County\tH1\n50249\t19187\tStratford\tIA\tWebster County\tH1\n50544\t19187\tHarcourt\tIA\tWebster County\tH1\n50524\t19187\tClare\tIA\tWebster County\tH1\n50566\t19187\tMoorland\tIA\tWebster County\tH1\n50591\t19187\tThor\tIA\tWebster County\tH1\n50217\t19187\tPaton\tIA\tWebster County\tH1\n50533\t19187\tEagle grove\tIA\tWebster County\tH1\n50569\t19187\tOtho\tIA\tWebster County\tH1\n50532\t19187\tDuncombe\tIA\tWebster County\tH1\n50523\t19187\tCallender\tIA\tWebster County\tH1\n50563\t19187\tManson\tIA\tWebster County\tH1\n50538\t19187\tFarnhamville\tIA\tWebster County\tH1\n50557\t19187\tLehigh\tIA\tWebster County\tH1\n50465\t19189\tRake\tIA\tWinnebago County\tH1\n50424\t19189\tBuffalo center\tIA\tWinnebago County\tH1\n50459\t19189\tNorthwood\tIA\tWinnebago County\tH1\n50453\t19189\tLeland\tIA\tWinnebago County\tH1\n50446\t19189\tJoice\tIA\tWinnebago County\tH1\n50444\t19189\tHanlontown\tIA\tWinnebago County\tH1\n50450\t19189\tLake mills\tIA\tWinnebago County\tH1\n50423\t19189\tBritt\tIA\tWinnebago County\tH1\n50473\t19189\tScarville\tIA\tWinnebago County\tH1\n50484\t19189\tWoden\tIA\tWinnebago County\tH1\n50434\t19189\tFertile\tIA\tWinnebago County\tH1\n50478\t19189\tThompson\tIA\tWinnebago County\tH1\n50436\t19189\tForest city\tIA\tWinnebago County\tH1\n52132\t19191\tCalmar\tIA\tWinneshiek County\tH1\n52172\t19191\tWaukon\tIA\tWinneshiek County\tH1\n52161\t19191\tOssian\tIA\tWinneshiek County\tH1\n52101\t19191\tDecorah\tIA\tWinneshiek County\tH1\n52136\t19191\tCresco\tIA\tWinneshiek County\tH1\n52162\t19191\tPostville\tIA\tWinneshiek County\tH1\n52168\t19191\tSpillville\tIA\tWinneshiek County\tH1\n52149\t19191\tHighlandville\tIA\tWinneshiek County\tH1\n52133\t19191\tCastalia\tIA\tWinneshiek County\tH1\n52165\t19191\tRidgeway\tIA\tWinneshiek County\tH1\n52144\t19191\tFort atkinson\tIA\tWinneshiek County\tH1\n52140\t19191\tDorchester\tIA\tWinneshiek County\tH1\n52171\t19191\tWaucoma\tIA\tWinneshiek County\tH1\n51006\t19193\tBattle creek\tIA\tWoodbury County\tH1\n51054\t19193\tSergeant bluff\tIA\tWoodbury County\tH1\n51106\t19193\tSioux city\tIA\tWoodbury County\tH1\n51109\t19193\tSioux city\tIA\tWoodbury County\tH1\n51108\t19193\tSioux city\tIA\tWoodbury County\tH1\n51048\t19193\tPierson\tIA\tWoodbury County\tH1\n51101\t19193\tSioux city\tIA\tWoodbury County\tH1\n51056\t19193\tSmithland\tIA\tWoodbury County\tH1\n51044\t19193\tOto\tIA\tWoodbury County\tH1\n51007\t19193\tBronson\tIA\tWoodbury County\tH1\n51039\t19193\tMoville\tIA\tWoodbury County\tH1\n51026\t19193\tHornick\tIA\tWoodbury County\tH1\n51063\t19193\tWhiting\tIA\tWoodbury County\tH1\n51015\t19193\tClimbing hill\tIA\tWoodbury County\tH1\n51028\t19193\tKingsley\tIA\tWoodbury County\tH1\n51055\t19193\tSloan\tIA\tWoodbury County\tH1\n51061\t19193\tWashta\tIA\tWoodbury County\tH1\n51034\t19193\tMapleton\tIA\tWoodbury County\tH1\n51111\t19193\tSioux city\tIA\tWoodbury County\tH1\n51052\t19193\tSalix\tIA\tWoodbury County\tH1\n51004\t19193\tAnthon\tIA\tWoodbury County\tH1\n51103\t19193\tSioux city\tIA\tWoodbury County\tH1\n51104\t19193\tSioux city\tIA\tWoodbury County\tH1\n51019\t19193\tDanbury\tIA\tWoodbury County\tH1\n51105\t19193\tSioux city\tIA\tWoodbury County\tH1\n51016\t19193\tCorrectionville\tIA\tWoodbury County\tH1\n51102\t19193\tSioux city\tIA\tWoodbury County\tH1\n51018\t19193\tCushing\tIA\tWoodbury County\tH1\n51030\t19193\tLawton\tIA\tWoodbury County\tH1\n50440\t19195\tGrafton\tIA\tWorth County\tH1\n50464\t19195\tPlymouth\tIA\tWorth County\tH1\n50426\t19195\tCarpenter\tIA\tWorth County\tH1\n50461\t19195\tOsage\tIA\tWorth County\tH1\n50456\t19195\tManly\tIA\tWorth County\tH1\n50401\t19195\tMason city\tIA\tWorth County\tH1\n50472\t19195\tSaint ansgar\tIA\tWorth County\tH1\n50459\t19195\tNorthwood\tIA\tWorth County\tH1\n50446\t19195\tJoice\tIA\tWorth County\tH1\n50444\t19195\tHanlontown\tIA\tWorth County\tH1\n50450\t19195\tLake mills\tIA\tWorth County\tH1\n50448\t19195\tKensett\tIA\tWorth County\tH1\n50434\t19195\tFertile\tIA\tWorth County\tH1\n50071\t19197\tDows\tIA\tWright County\tH1\n50525\t19197\tClarion\tIA\tWright County\tH1\n50447\t19197\tKanawha\tIA\tWright County\tH1\n50034\t19197\tBlairsburg\tIA\tWright County\tH1\n50595\t19197\tWebster city\tIA\tWright County\tH1\n50599\t19197\tWoolstock\tIA\tWright County\tH1\n50271\t19197\tWilliams\tIA\tWright County\tH1\n50470\t19197\tRowan\tIA\tWright County\tH1\n50542\t19197\tGoldfield\tIA\tWright County\tH1\n50577\t19197\tRenwick\tIA\tWright County\tH1\n50006\t19197\tAlden\tIA\tWright County\tH1\n50420\t19197\tAlexander\tIA\tWright County\tH1\n50421\t19197\tBelmond\tIA\tWright County\tH1\n50533\t19197\tEagle grove\tIA\tWright County\tH1\n50532\t19197\tDuncombe\tIA\tWright County\tH1\n50457\t19197\tMeservey\tIA\tWright County\tH1\n50430\t19197\tCorwith\tIA\tWright County\tH1\n50101\t19197\tGalt\tIA\tWright County\tH1\n66749\t20001\tIola\tKS\tAllen County\tH1\n66742\t20001\tGas\tKS\tAllen County\tH1\n66748\t20001\tHumboldt\tKS\tAllen County\tH1\n66039\t20001\tKincaid\tKS\tAllen County\tH1\n66732\t20001\tElsmore\tKS\tAllen County\tH1\n66758\t20001\tNeosho falls\tKS\tAllen County\tH1\n66015\t20001\tColony\tKS\tAllen County\tH1\n66751\t20001\tLa harpe\tKS\tAllen County\tH1\n66720\t20001\tChanute\tKS\tAllen County\tH1\n66755\t20001\tMoran\tKS\tAllen County\tH1\n66772\t20001\tSavonburg\tKS\tAllen County\tH1\n66716\t20001\tBronson\tKS\tAllen County\tH1\n66014\t20003\tCenterville\tKS\tAnderson County\tH1\n66749\t20003\tIola\tKS\tAnderson County\tH1\n66033\t20003\tGreeley\tKS\tAnderson County\tH1\n66032\t20003\tGarnett\tKS\tAnderson County\tH1\n66093\t20003\tWestphalia\tKS\tAnderson County\tH1\n66080\t20003\tRichmond\tKS\tAnderson County\tH1\n66091\t20003\tWelda\tKS\tAnderson County\tH1\n66010\t20003\tBlue mound\tKS\tAnderson County\tH1\n66039\t20003\tKincaid\tKS\tAnderson County\tH1\n66095\t20003\tWilliamsburg\tKS\tAnderson County\tH1\n66758\t20003\tNeosho falls\tKS\tAnderson County\tH1\n66015\t20003\tColony\tKS\tAnderson County\tH1\n66058\t20005\tMuscotah\tKS\tAtchison County\tH1\n66023\t20005\tEffingham\tKS\tAtchison County\tH1\n66424\t20005\tEverest\tKS\tAtchison County\tH1\n66016\t20005\tCummings\tKS\tAtchison County\tH1\n66552\t20005\tWhiting\tKS\tAtchison County\tH1\n66041\t20005\tLancaster\tKS\tAtchison County\tH1\n66088\t20005\tValley falls\tKS\tAtchison County\tH1\n66002\t20005\tAtchison\tKS\tAtchison County\tH1\n66436\t20005\tHolton\tKS\tAtchison County\tH1\n66439\t20005\tHorton\tKS\tAtchison County\tH1\n66060\t20005\tNortonville\tKS\tAtchison County\tH1\n67104\t20007\tMedicine lodge\tKS\tBarber County\tH1\n67009\t20007\tAttica\tKS\tBarber County\tH1\n67112\t20007\tNashville\tKS\tBarber County\tH1\n67138\t20007\tSharon\tKS\tBarber County\tH1\n67134\t20007\tSawyer\tKS\tBarber County\tH1\n67061\t20007\tHazelton\tKS\tBarber County\tH1\n67028\t20007\tCoats\tKS\tBarber County\tH1\n67071\t20007\tLake city\tKS\tBarber County\tH1\n67070\t20007\tKiowa\tKS\tBarber County\tH1\n67057\t20007\tHardtner\tKS\tBarber County\tH1\n67143\t20007\tSun city\tKS\tBarber County\tH1\n67065\t20007\tIsabel\tKS\tBarber County\tH1\n67665\t20009\tRussell\tKS\tBarton County\tH1\n67450\t20009\tHolyrood\tKS\tBarton County\tH1\n67564\t20009\tOlmitz\tKS\tBarton County\tH1\n67526\t20009\tEllinwood\tKS\tBarton County\tH1\n67511\t20009\tAlbert\tKS\tBarton County\tH1\n67525\t20009\tClaflin\tKS\tBarton County\tH1\n67427\t20009\tBushton\tKS\tBarton County\tH1\n67565\t20009\tOtis\tKS\tBarton County\tH1\n67544\t20009\tHoisington\tKS\tBarton County\tH1\n67530\t20009\tGreat bend\tKS\tBarton County\tH1\n67567\t20009\tPawnee rock\tKS\tBarton County\tH1\n66738\t20011\tFulton\tKS\tBourbon County\tH1\n66746\t20011\tHepler\tKS\tBourbon County\tH1\n66741\t20011\tGarland\tKS\tBourbon County\tH1\n66701\t20011\tFort scott\tKS\tBourbon County\tH1\n66711\t20011\tArcadia\tKS\tBourbon County\tH1\n66775\t20011\tStark\tKS\tBourbon County\tH1\n66754\t20011\tMapleton\tKS\tBourbon County\tH1\n66010\t20011\tBlue mound\tKS\tBourbon County\tH1\n66779\t20011\tUniontown\tKS\tBourbon County\tH1\n66769\t20011\tRedfield\tKS\tBourbon County\tH1\n66056\t20011\tMound city\tKS\tBourbon County\tH1\n66780\t20011\tWalnut\tKS\tBourbon County\tH1\n66755\t20011\tMoran\tKS\tBourbon County\tH1\n66772\t20011\tSavonburg\tKS\tBourbon County\tH1\n66716\t20011\tBronson\tKS\tBourbon County\tH1\n66094\t20013\tWhite cloud\tKS\tBrown County\tH1\n66017\t20013\tDenton\tKS\tBrown County\tH1\n66424\t20013\tEverest\tKS\tBrown County\tH1\n66534\t20013\tSabetha\tKS\tBrown County\tH1\n66041\t20013\tLancaster\tKS\tBrown County\tH1\n66434\t20013\tHiawatha\tKS\tBrown County\tH1\n66516\t20013\tNetawaka\tKS\tBrown County\tH1\n66527\t20013\tPowhattan\tKS\tBrown County\tH1\n66515\t20013\tMorrill\tKS\tBrown County\tH1\n66439\t20013\tHorton\tKS\tBrown County\tH1\n66532\t20013\tRobinson\tKS\tBrown County\tH1\n66425\t20013\tFairview\tKS\tBrown County\tH1\n66550\t20013\tWetmore\tKS\tBrown County\tH1\n67042\t20015\tEl dorado\tKS\tButler County\tH1\n67132\t20015\tRosalia\tKS\tButler County\tH1\n67144\t20015\tTowanda\tKS\tButler County\tH1\n67072\t20015\tLatham\tKS\tButler County\tH1\n67002\t20015\tAndover\tKS\tButler County\tH1\n67008\t20015\tAtlanta\tKS\tButler County\tH1\n66842\t20015\tCassoday\tKS\tButler County\tH1\n67232\t20015\tWichita\tKS\tButler County\tH1\n67010\t20015\tAugusta\tKS\tButler County\tH1\n67045\t20015\tEureka\tKS\tButler County\tH1\n67230\t20015\tWichita\tKS\tButler County\tH1\n67039\t20015\tDouglass\tKS\tButler County\tH1\n67017\t20015\tBenton\tKS\tButler County\tH1\n67114\t20015\tNewton\tKS\tButler County\tH1\n67074\t20015\tLeon\tKS\tButler County\tH1\n67133\t20015\tRose hill\tKS\tButler County\tH1\n67228\t20015\tWichita\tKS\tButler County\tH1\n66840\t20015\tBurns\tKS\tButler County\tH1\n67154\t20015\tWhitewater\tKS\tButler County\tH1\n67041\t20015\tElbing\tKS\tButler County\tH1\n67123\t20015\tPotwin\tKS\tButler County\tH1\n67012\t20015\tBeaumont\tKS\tButler County\tH1\n66869\t20017\tStrong city\tKS\tChase County\tH1\n66845\t20017\tCottonwood falls\tKS\tChase County\tH1\n66862\t20017\tMatfield green\tKS\tChase County\tH1\n66850\t20017\tElmdale\tKS\tChase County\tH1\n66840\t20017\tBurns\tKS\tChase County\tH1\n66843\t20017\tCedar point\tKS\tChase County\tH1\n66858\t20017\tLincolnville\tKS\tChase County\tH1\n66801\t20017\tEmporia\tKS\tChase County\tH1\n66865\t20017\tOlpe\tKS\tChase County\tH1\n67344\t20019\tElk city\tKS\tChautauqua County\tH1\n67353\t20019\tMoline\tKS\tChautauqua County\tH1\n67346\t20019\tGrenola\tKS\tChautauqua County\tH1\n67355\t20019\tNiotaze\tKS\tChautauqua County\tH1\n67334\t20019\tChautauqua\tKS\tChautauqua County\tH1\n67347\t20019\tHavana\tKS\tChautauqua County\tH1\n67024\t20019\tCedar vale\tKS\tChautauqua County\tH1\n67349\t20019\tHoward\tKS\tChautauqua County\tH1\n67361\t20019\tSedan\tKS\tChautauqua County\tH1\n67352\t20019\tLongton\tKS\tChautauqua County\tH1\n67360\t20019\tPeru\tKS\tChautauqua County\tH1\n67336\t20021\tChetopa\tKS\tCherokee County\tH1\n66739\t20021\tGalena\tKS\tCherokee County\tH1\n66724\t20021\tCherokee\tKS\tCherokee County\tH1\n66773\t20021\tScammon\tKS\tCherokee County\tH1\n66725\t20021\tColumbus\tKS\tCherokee County\tH1\n66713\t20021\tBaxter springs\tKS\tCherokee County\tH1\n66762\t20021\tPittsburg\tKS\tCherokee County\tH1\n67356\t20021\tOswego\tKS\tCherokee County\tH1\n66728\t20021\tCrestline\tKS\tCherokee County\tH1\n66770\t20021\tRiverton\tKS\tCherokee County\tH1\n66781\t20021\tWeir\tKS\tCherokee County\tH1\n66753\t20021\tMc cune\tKS\tCherokee County\tH1\n66778\t20021\tTreece\tKS\tCherokee County\tH1\n66782\t20021\tWest mineral\tKS\tCherokee County\tH1\n67741\t20023\tKanorado\tKS\tCheyenne County\tH1\n67756\t20023\tSaint francis\tKS\tCheyenne County\tH1\n67731\t20023\tBird city\tKS\tCheyenne County\tH1\n67834\t20025\tBucklin\tKS\tClark County\tH1\n67127\t20025\tProtection\tKS\tClark County\tH1\n67842\t20025\tFord\tKS\tClark County\tH1\n67844\t20025\tFowler\tKS\tClark County\tH1\n67865\t20025\tMinneola\tKS\tClark County\tH1\n67840\t20025\tEnglewood\tKS\tClark County\tH1\n67831\t20025\tAshland\tKS\tClark County\tH1\n67410\t20027\tAbilene\tKS\tClay County\tH1\n67466\t20027\tMiltonvale\tKS\tClay County\tH1\n67447\t20027\tGreen\tKS\tClay County\tH1\n66937\t20027\tClifton\tKS\tClay County\tH1\n67458\t20027\tLongford\tKS\tClay County\tH1\n67468\t20027\tMorganville\tKS\tClay County\tH1\n66962\t20027\tPalmer\tKS\tClay County\tH1\n66938\t20027\tClyde\tKS\tClay County\tH1\n67432\t20027\tClay center\tKS\tClay County\tH1\n67487\t20027\tWakefield\tKS\tClay County\tH1\n66935\t20029\tBelleville\tKS\tCloud County\tH1\n66901\t20029\tConcordia\tKS\tCloud County\tH1\n66966\t20029\tScandia\tKS\tCloud County\tH1\n67455\t20029\tLincoln\tKS\tCloud County\tH1\n66940\t20029\tCuba\t
